vi "CheckFreeErrorCount.vi"(8 "ErrorIn":errorcluster caption="Error In(no Error)", 10 "Library":string, 11 "ReferenceIn":refnum<class "ErrorDefinitionSQLite.lvclass"> caption="Reference In") -> (0 "ErrorOut":errorcluster caption="Error Out", 2 "FreeErrorsInLibrary":i32, 3 "ReferenceOut":refnum<class "ErrorDefinitionSQLite.lvclass"> caption="Reference Out")   [LabVIEW 2018, in "ErrorDefinitionSQLite.lvclass"]
uses:
  ErrorDefinitionSQLite.lvclass
  <vilib>/drjdpowell/SQLite Library/SQL Connection/Execute SQL.vi
  <vilib>/drjdpowell/SQLite Library/SQLite.lvlib
  <vilib>/drjdpowell/SQLite Library/SQL Connection/Connection.lvclass
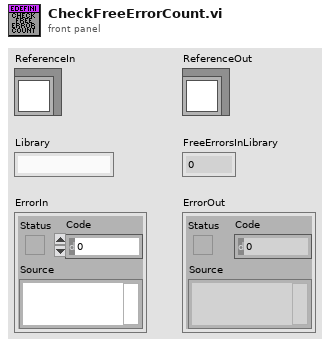
[diagram p1: front panel]
types:
  T1 = typedef "ErrorDefinitionSQLite.lvclass/ObjectAttributes.ctl" = cluster{"Path":path, "SQLiteRef":refnum<class "Connection.lvclass">, "EndOfRange":i32, "DefaultLibrarySize":i32, "StartOfRange":i32}
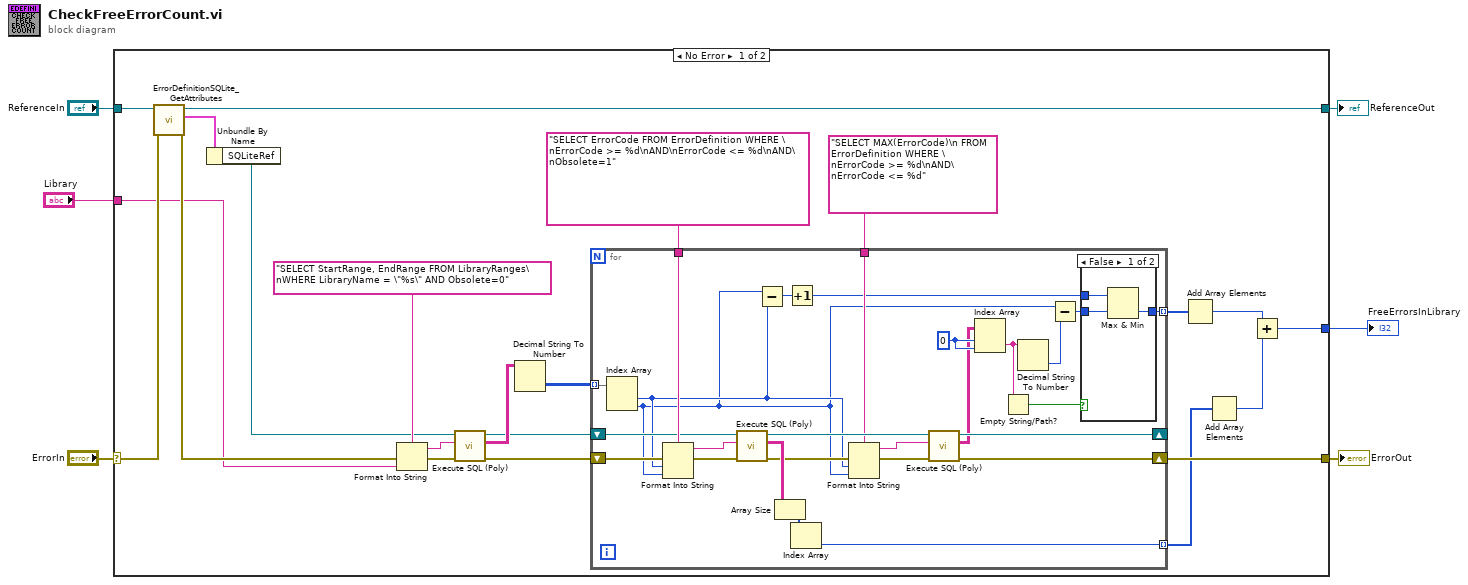
[diagram p0: block diagram]
diagram:
  n1 = case shown="No Error" "ErrorIn" {
    selector: "ErrorIn" -> [w28 w61]
    tunnel: [w15 w61] -> w5
    tunnel: [w26 w60] -> w3
    tunnel: "ReferenceIn" -> [w27 w60]
    tunnel: "Library" -> [w14 _]
    tunnel: [w8 _] -> w1
    frame No Error {
      n2 = call "ErrorDefinitionSQLite_GetAttributes.vi"("ErrorIn"=w28, "Reference in"=w27) -> ("ErrorOut"=w16:errorcluster, "Data"=w25:T1, "Reference out"=w26:refnum<class "ErrorDefinitionSQLite.lvclass">)  [unwired: 6 in, 1 out]
      n3 = Unbundle By Name(w25) -> ("SQLiteRef"=w13:refnum<class "Connection.lvclass">)
      n4 = Format Into String(format string="SELECT StartRange, EndRange FROM LibraryRanges\nWHERE LibraryName = \"%s\" AND Obsolete=0" ("SQL"), error in=w16, w14) -> (resulting string=w22:string, error out=w19:errorcluster)  [unwired: 1 in]
      n5 = call-poly <vilib>:"Execute SQL (Poly).vi"("error in (no error)"=w19, "SQL"=w22, "SQLite Connection in"=w13) -> ("error out"=w20:errorcluster, "Result Set"=w23:string[][], "SQLite Connection"=w21:refnum<class "Connection.lvclass">)  [unwired: 5 in, 1 out]
      n6 = Decimal String To Number(string=w23) -> (number=w24:i32[][])  [unwired: 2 in, 1 out]
      n7 = for {
        tunnel: "SELECT ErrorCode FROM ErrorDefinition WHERE \nErrorCode >= %d\nAND\nErrorCode <= %d\nAND\nObsolete=1" ("SQL") -> [w53]
        shift-right: [w42] -> w15
        shift-left: w20 -> [w52]
        shift-right: [w43] -> _
        shift-left: w21 -> [w51]
        tunnel: w24 -> [w50] mode=indexing
        tunnel: [w47] -> w12 mode=indexing
        tunnel: "SELECT MAX(ErrorCode)\n FROM ErrorDefinition WHERE \nErrorCode >= %d\nAND\nErrorCode <= %d" ("SQL") -> [w40]
        tunnel: [w33] -> w9 mode=indexing
        w44 = 0 ("index (row)")
        n8 = Index Array(array=w50) -> (element #1=w38:i32, element #2=w36:i32)  [unwired: 2 in]
        n9 = Format Into String(format string=w53, error in=w52, w38, w36) -> (resulting string=w54:string, error out=w55:errorcluster)  [unwired: 1 in]
        n10 = call-poly <vilib>:"Execute SQL (Poly).vi"("error in (no error)"=w55, "SQL"=w54, "SQLite Connection in"=w51) -> ("error out"=w45:errorcluster, "Result Set"=w49:string[][], "SQLite Connection"=w46:refnum<class "Connection.lvclass">)  [unwired: 5 in, 1 out]
        n11 = Subtract(x=w36, y=w38) -> (x-y=w34:i32)
        n12 = Array Size(array=w49) -> (size(s)=w48:i32[])
        n13 = Increment(x=w34) -> (x+1=w32:i32)
        n14 = Index Array(array=w48) -> (element=w47:i32)  [unwired: 1 in]
        n15 = Format Into String(format string=w40, error in=w45, w38, w36) -> (resulting string=w39:string, error out=w41:errorcluster)  [unwired: 1 in]
        n16 = call-poly <vilib>:"Execute SQL (Poly).vi"("error in (no error)"=w41, "SQL"=w39, "SQLite Connection in"=w46) -> ("error out"=w42:errorcluster, "Result Set"=w31:string[][], "SQLite Connection"=w43:refnum<class "Connection.lvclass">)  [unwired: 5 in, 1 out]
        n17 = Index Array(array=w31, index (row)=w44, index (col)=w44) -> (element=w29:string)
        n18 = Empty String/Path?(string/path=w29) -> (empty?=w30:bool)
        n19 = Decimal String To Number(string=w29) -> (number=w37:i32)  [unwired: 2 in, 1 out]
        n20 = Subtract(x=w36, y=w37) -> (x-y=w35:i32)
        n21 = case shown="False" w30 {
          tunnel: w35 -> [w58 _]
          tunnel: [w57 w59] -> w33
          tunnel: w32 -> [w56 w59]
          frame False {
            n22 = Max & Min(x=w56, y=w58) -> (min(x,y)=w57:i32)  [unwired: 1 out]
          }
          frame True {
          }
        }
      }
      n23 = Add Array Elements(numeric array=w9) -> (sum=w7:i32)
      n24 = Add Array Elements(numeric array=w12) -> (sum=w11:i32)
      n25 = Add(x=w7, y=w11) -> (x+y=w8:i32)
    }
    frame Error {
    }
  }
  "ErrorOut" <- w5
  "ReferenceOut" <- w3
  "FreeErrorsInLibrary" <- w1
